vi "Player Info.vi"(11 "Trek in":refnum<class "Trek.lvclass">) -> (0 "Defeat Speech":string, 1 "Victory Speech":string, 2 "Name":string, 3 "Trek out":refnum<class "Trek.lvclass">)   [LabVIEW 2015, in "Trek.lvclass"]
uses:
  Trek.lvclass
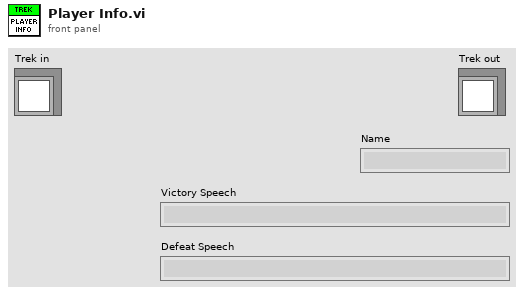
[diagram p1: front panel]
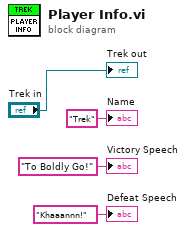
[diagram p0: block diagram]
diagram:
  "Trek out" <- "Trek in"
  "Name" <- "Trek" ("Name")
  "Victory Speech" <- "To Boldly Go!" ("Victory Speech")
  "Defeat Speech" <- "Khaaannn!" ("Defeat Speech")
